vi "Init Vecto.vi"(8 "error in (no error)":errorcluster, 11 "VolatusCoreTask in":refnum<class "VolatusCoreTask.lvclass">) -> (0 "error out":errorcluster, 3 "VolatusCoreTask out":refnum<class "VolatusCoreTask.lvclass">)   [LabVIEW 2020, in "Volatus.lvlib" / "VolatusCoreTask.lvclass"]
uses:
  VolatusCoreTask.lvclass
  VolatusCoreTask.lvclass/VolatusCoreTask.ctl
  lv-vecto/Vecto/Vecto/Vecto.lvclass
  lv-vecto/Vecto/EventLogHandler/EventLogHandler.lvclass
  lv-vecto/Vecto/Init Implementations.ctl
  lv-vecto/Vecto/Vecto.lvlib
  VectoEventBridge/VectoEventBridge.lvclass
  App/App.lvclass
  C:/dev/lv20CE/relink/lv-volatus/Volatus/VectoEventBridge/VectoEventBridge.lvclass
  C:/dev/lv20CE/relink/lv-vecto/Vecto/EventLogHandler/EventLogHandler.lvclass
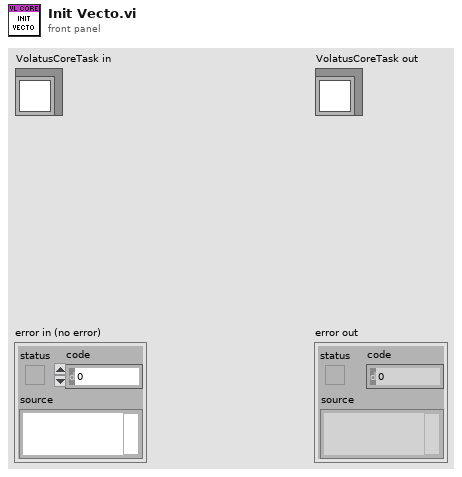
[diagram p1: front panel]
types:
  T1 = typedef "Vecto.lvlib/Init Implementations.ctl" = cluster{"EventLogger":refnum<class "EventLogHandler.lvclass">}
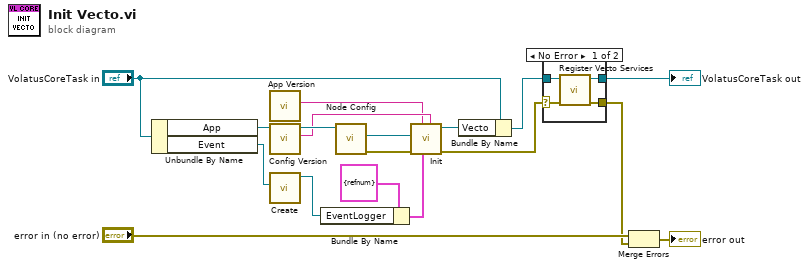
[diagram p0: block diagram]
diagram:
  n1 = Unbundle By Name("VolatusCoreTask in") -> ("App"=w11:refnum<class "App.lvclass">, "Event"=w14:refnum<class "EventAPI.lvclass">)
  n2 = call "App Version.vi"() -> ("App Version"=w8:string)  [unwired: 11 in]
  n3 = call "Config Version.vi"("App in"=w11) -> ("Cfg Version"=w9:string, "App out"=w10:refnum<class "App.lvclass">)  [unwired: 8 in, 1 out]
  n4 = call "Create.vi"("EventAPI"=w14) -> ("VectoEventBridge out"=w12:refnum<class "VectoEventBridge.lvclass">)  [unwired: 9 in, 1 out]
  n5 = Bundle By Name(cluster=T1 {"EventLogger"=refnum} ("Init Implementations"), "EventLogger"=w12) -> (w13:T1)
  n6 = call-dynamic "Node Config.vi"("App in"=w10) -> ("error out"=w17:errorcluster, "Node Config"=w16:refnum<class "Node Config.lvclass">)  [unwired: 8 in, 1 out]
  n7 = call "Init.vi"("Config Version"=w9, "Init Implementations"=w13, "App Version"=w8, "error in (no error)"=w17, "Node"=w16) -> ("error out"=w3:errorcluster, "Vecto out"=w7:refnum<class "Vecto.lvclass">)  [unwired: 5 in]
  n8 = Bundle By Name(cluster="VolatusCoreTask in", "Vecto"=w7) -> (w5:refnum<class "VolatusCoreTask.lvclass">)
  n9 = case shown="No Error" w3 {
    selector: w3 -> [w20 w24]
    tunnel: w5 -> [w22 w23]
    tunnel: [w21 w23] -> w4
    tunnel: [w19 w24] -> w1
    frame No Error {
      n10 = call "Register Vecto Services.vi"("error in (no error)"=w20, "VolatusCoreTask in"=w22) -> ("error out"=w19:errorcluster, "VolatusCoreTask out"=w21:refnum<class "VolatusCoreTask.lvclass">)  [unwired: 8 in]
    }
    frame Error {
    }
  }
  "VolatusCoreTask out" <- w4
  n11 = Merge Errors("error in (no error)", w1) -> (→"error out":errorcluster)
